vi "Display Item Info.vi"(8 "error in (no error)":errorcluster, 9 "Config":T1, 10 "Control References":T5, 11 "VI in":refnum<class "VI.lvclass">) -> (0 "error out":errorcluster, 3 "VI out":refnum<class "VI.lvclass">)   [LabVIEW 2020, in "VI Properties Editor.lvlib" / "VI.lvclass"]
doc: "Displays the data of <B>VI in</B> to the controls identified by <B>Control References</B>, taking into account <B>Config</B>."
uses:
  VI.lvclass
  C:/Users/acasalen/Documents/LabVIEW Data/Projects/VI-Properties-Editor/source/Classes/Item/Item.lvclass
  <vilib>/LabVIEW Icon API/lv_icon/Classes/Icon/Icon.lvclass
  Control/Control.lvclass
  VI Properties Editor.lvlib
  <vilib>/LabVIEW Icon API/LabVIEW Icon API.lvlib
  CTLs/Main References.ctl
  CTLs/Filter Column.ctl
  CTLs/Filter Type.ctl
  CTLs/Filter Info.ctl
  CTLs/Config.ctl
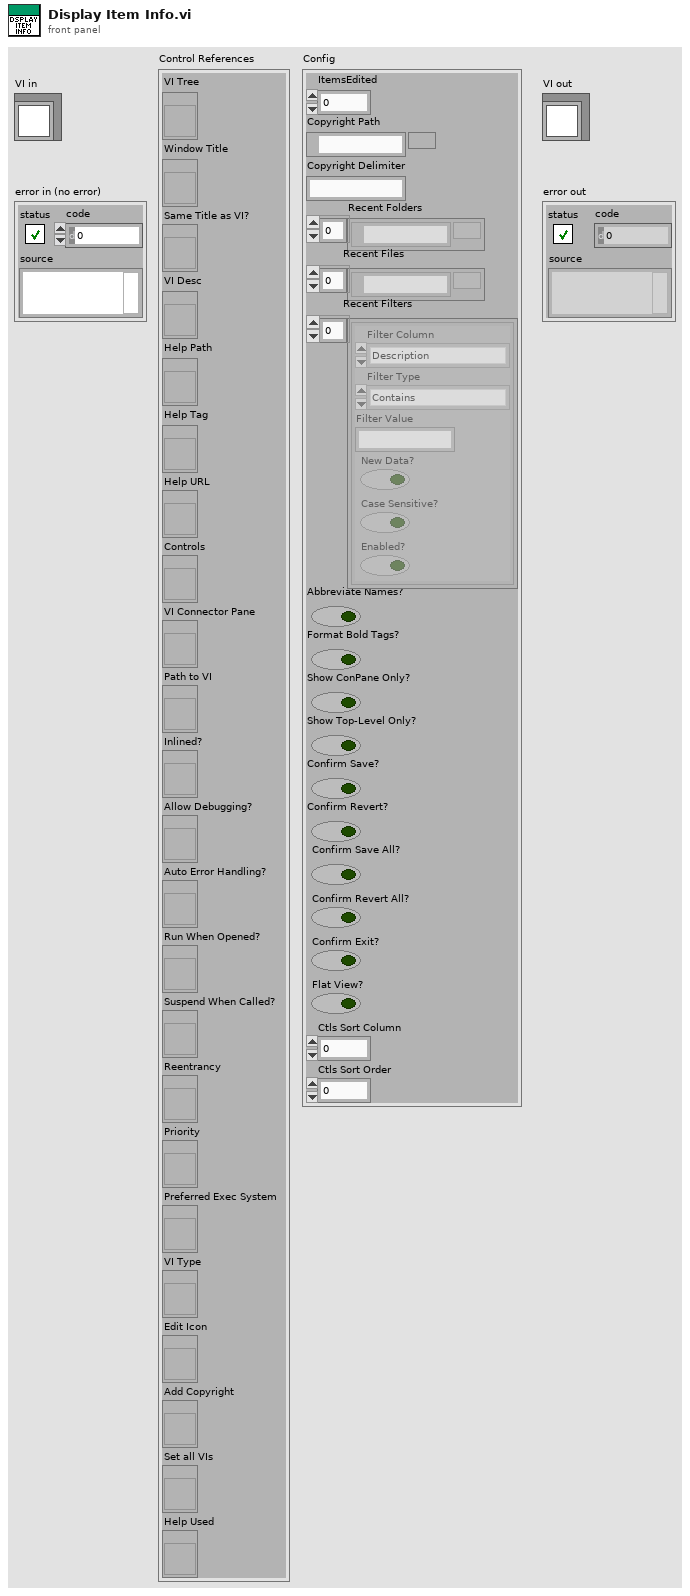
[diagram p1: front panel]
types:
  T1 = typedef "VI Properties Editor.lvlib/Config.ctl" = cluster{"ItemsEdited":u32, "Copyright Path":path, "Copyright Delimiter":string, "Recent Folders":path[], "Recent Files":path[], "Recent Filters":T2[], "Abbreviate Names?":bool, "Format Bold Tags?":bool, "Show ConPane Only?":bool, "Show Top-Level Only?":bool, "Confirm Save?":bool, "Confirm Revert?":bool, "Confirm Save All?":bool, "Confirm Revert All?":bool, "Confirm Exit?":bool, "Flat View?":bool, "Ctls Sort Column":i32, "Ctls Sort Order":i32}
  T2 = typedef "VI Properties Editor.lvlib/Filter Info.ctl" = cluster{"Filter Column":T3, "Filter Type":T4, "Filter Value":string, "New Data?":bool, "Case Sensitive?":bool, "Enabled?":bool}
  T3 = typedef "VI Properties Editor.lvlib/Filter Column.ctl" = enum16{"Name", "Path", "Type", "Window Title", "Description", "Help Path", "Help Tag", "Custom Title?", "Reentrancy", "Inlined?", "Help URL", "Help Type", "Allow Debugging?", "Auto Error Handling?", "Run When Opened?", "Suspend When Called?", "Priority", "Preferred Exec Sytem", "Control Label", "Control Caption", "Control Description", "Control Tip Strip"}
  T4 = typedef "VI Properties Editor.lvlib/Filter Type.ctl" = enum16{"Contains", "Equals", "Starts with", "Ends with", "Is empty", "Does not contain", "Does not equal", "Is not empty"}
  T5 = typedef "VI Properties Editor.lvlib/Main References.ctl" = cluster{"VI Tree":refnum<vi>, "Window Title":refnum<vi>, "Same Title as VI?":refnum<vi>, "VI Desc":refnum<vi>, "Help Path":refnum<vi>, "Help Tag":refnum<vi>, "Help URL":refnum<vi>, "Controls":refnum<vi>, "VI Connector Pane":refnum<vi>, "Path to VI":refnum<vi>, "Inlined?":refnum<vi>, "Allow Debugging?":refnum<vi>, "Auto Error Handling?":refnum<vi>, "Run When Opened?":refnum<vi>, "Suspend When Called?":refnum<vi>, "Reentrancy":refnum<vi>, "Priority":refnum<vi>, "Preferred Exec System":refnum<vi>, "VI Type":refnum<vi>, "Edit Icon":refnum<vi>, "Add Copyright":refnum<vi>, "Set all VIs":refnum<vi>, "Help Used":refnum<vi>}
  T6 = typedef "imagedata.ctl" = cluster{"image type":i32, "image depth":i32, "image":u8[], "mask":u8[], "colors":u32[], "Rectangle":cluster{"left":i16, "top":i16, "right":i16, "bottom":i16}}
  T7 = enum32{"invalid execution system", "user interface", "standard", "instrument i/o", "data acquisition", "other 1", "other 2", "same as caller"}
  T8 = enum32{"invalid VI type", "Standard VI", "Control VI", "Global VI", "Polymorphic VI", "Configuration VI", "SubSystem", "Facade VI", "Method VI", "Statechart Diagram VI"}
  T9 = enum32{"invalid priority", "background priority", "normal priority", "above normal priority", "high priority", "time critical priority", "subroutine"}
  T10 = enum16{"Share clones between instances", "Preallocate clone for each instance"}
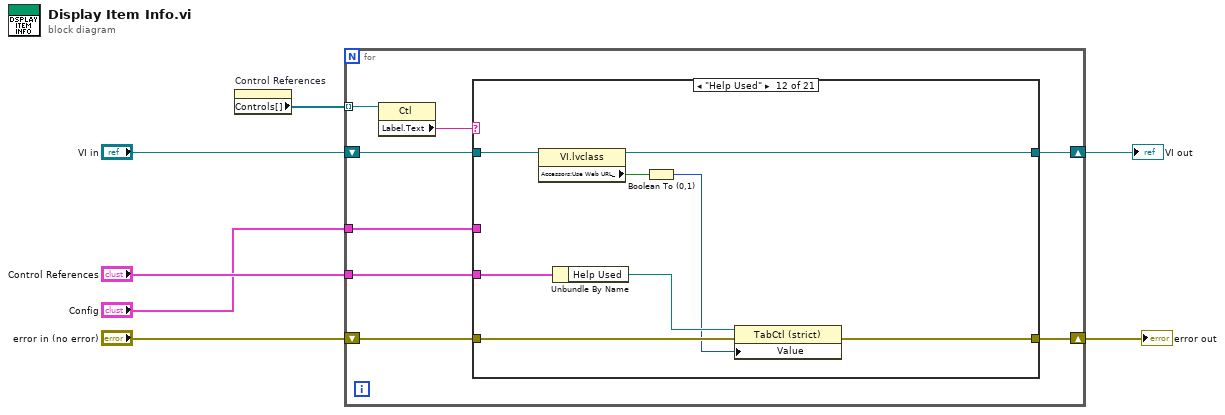
[diagram p0: block diagram]
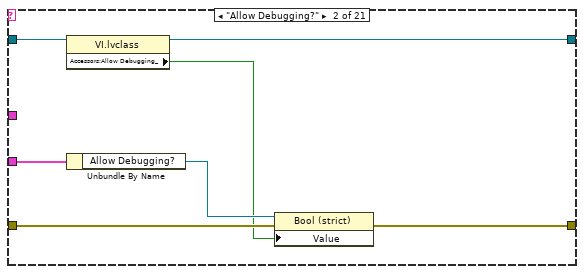
[diagram p3: hidden frame]
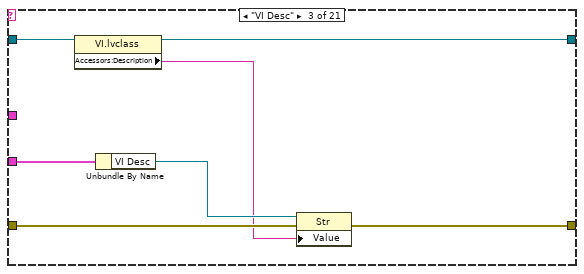
[diagram p4: hidden frame]
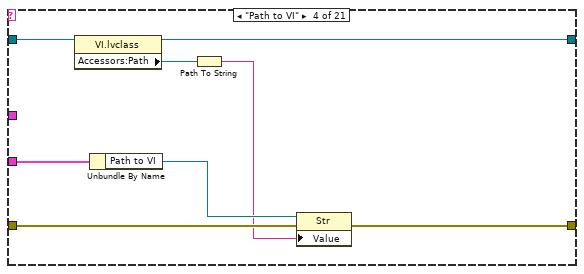
[diagram p5: hidden frame]
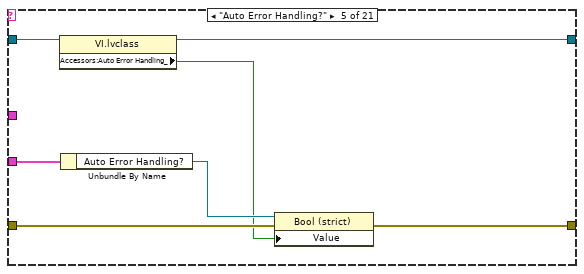
[diagram p6: hidden frame]
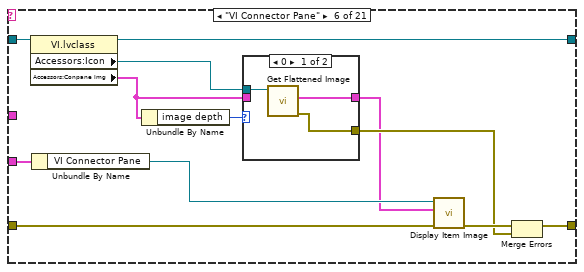
[diagram p7: hidden frame]
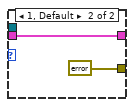
[diagram p8: hidden frame]
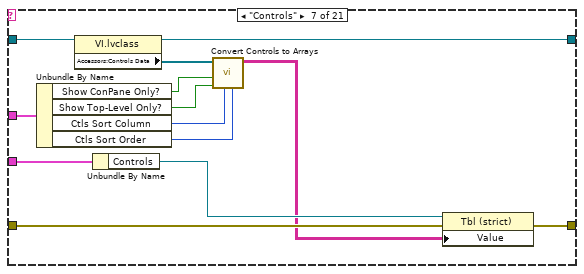
[diagram p9: hidden frame]
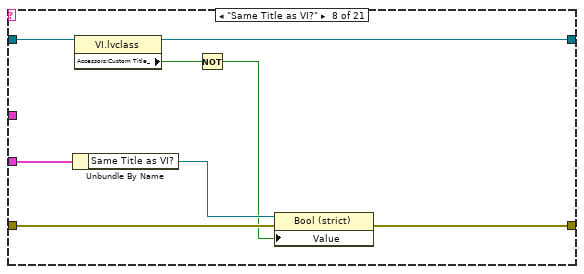
[diagram p10: hidden frame]
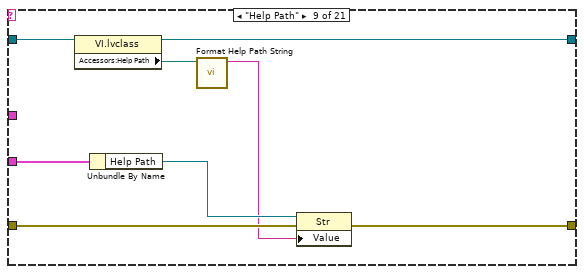
[diagram p11: hidden frame]
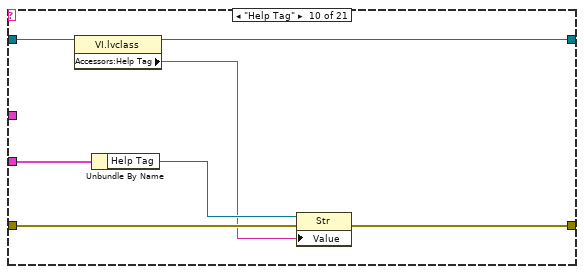
[diagram p12: hidden frame]
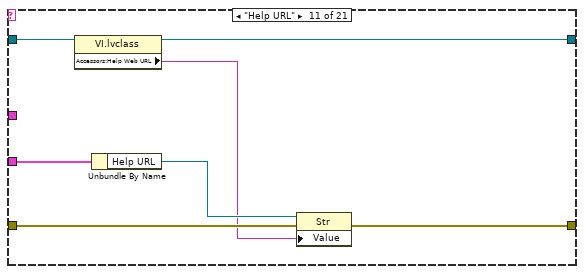
[diagram p13: hidden frame]
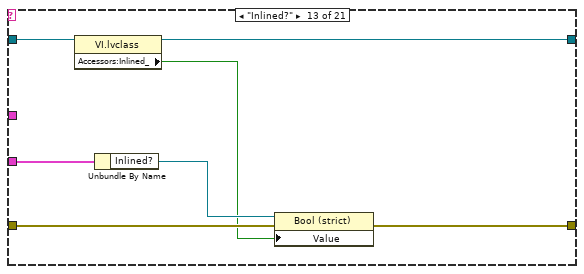
[diagram p14: hidden frame]
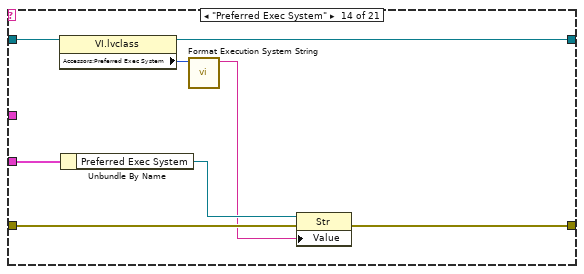
[diagram p15: hidden frame]
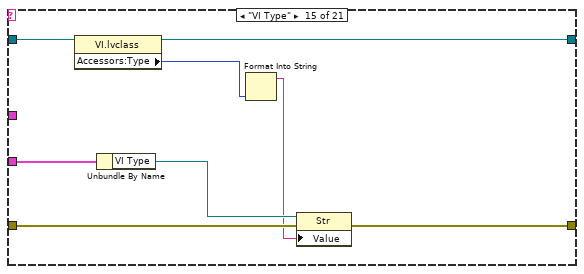
[diagram p16: hidden frame]
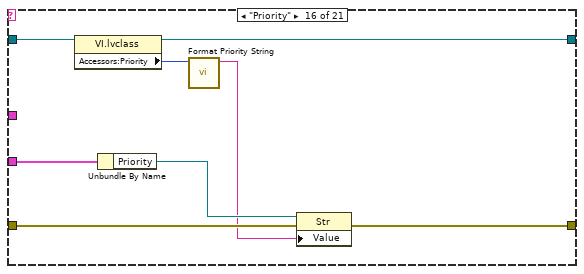
[diagram p17: hidden frame]
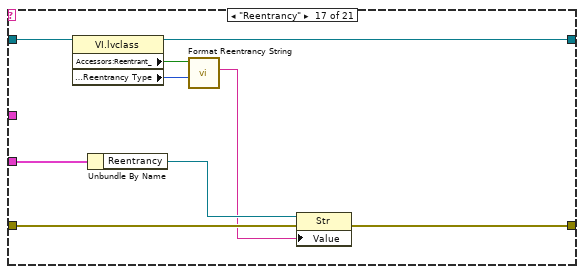
[diagram p18: hidden frame]
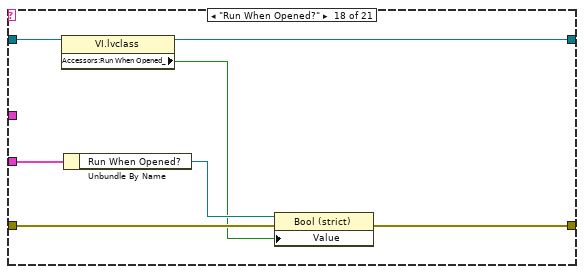
[diagram p19: hidden frame]
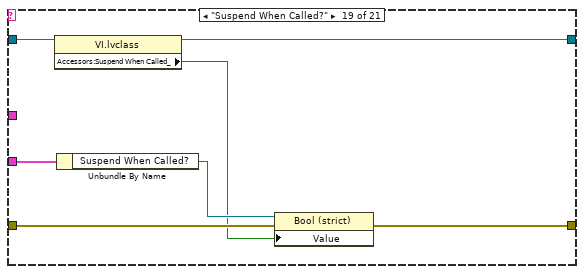
[diagram p20: hidden frame]
diagram:
  n1 = property on="Control References" class="Clust (strict)"() -> ("Controls[]"=w5:refnum<vi>[])  [unwired: 2 in, 2 out]
  n2 = for {
    shift-right: [w14] -> w6
    shift-left: "VI in" -> [w15]
    tunnel: w5 -> [w12] mode=indexing
    shift-right: [w10] -> w2
    shift-left: "error in (no error)" -> [w13]
    tunnel: "Control References" -> [w11]
    tunnel: "Config" -> [w9]
    n3 = property class="Ctl"(reference=w12) -> ("Label.Text"=w8:string)  [unwired: 1 in, 2 out]
    n4 = case shown="\"Help Used\"" w8 {
      tunnel: w15 -> [w17 w24 w31 w39 w46 w58 w76 w84 w92 w99 w106 w114 w121 w129 w137 w145 w154 w161 w168 w175 w177]
      tunnel: [w17 w23 w30 w38 w45 w57 w75 w83 w91 w98 w105 w113 w120 w128 w136 w144 w153 w160 w167 w174 w177] -> w14
      tunnel: w13 -> [w16 w20 w27 w35 w42 w49 w72 w80 w88 w95 w102 w110 w117 w125 w133 w141 w150 w157 w164 w171 w176]
      tunnel: w11 -> [_ w22 w29 w37 w44 w56 w74 w82 w90 w97 w104 w112 w119 w127 w135 w143 w152 w159 w166 w173 _]
      tunnel: [w16 w18 w25 w33 w40 w51 w71 w79 w87 w94 w101 w109 w116 w124 w132 w140 w149 w156 w163 w170 w176] -> w10
      tunnel: w9 -> [_ _ _ _ _ _ w69 _ _ _ _ _ _ _ _ _ _ _ _ _ _]
      frame Default {
      }
      frame "Allow Debugging?" {
        n5 = property class="VI.lvclass"(reference=w24) -> (reference out=w23:refnum<class "VI.lvclass">, "Accessors:Allow Debugging_"=w19:bool)  [unwired: 1 in, 1 out]
        n6 = Unbundle By Name(w22) -> ("Allow Debugging?"=w21:refnum<vi>)
        n7 = property class="Bool (strict)"(reference=w21, error in=w20, "Value"=w19) -> (error out=w18:errorcluster)  [unwired: 1 out]
      }
      frame "VI Desc" {
        n8 = property class="VI.lvclass"(reference=w31) -> (reference out=w30:refnum<class "VI.lvclass">, "Accessors:Description"=w26:string)  [unwired: 1 in, 1 out]
        n9 = Unbundle By Name(w29) -> ("VI Desc"=w28:refnum<vi>)
        n10 = property class="Str"(reference=w28, error in=w27, "Value"=w26) -> (error out=w25:errorcluster)  [unwired: 1 out]
      }
      frame "Path to VI" {
        n11 = property class="VI.lvclass"(reference=w39) -> (reference out=w38:refnum<class "VI.lvclass">, "Accessors:Path"=w34:path)  [unwired: 1 in, 1 out]
        n12 = Unbundle By Name(w37) -> ("Path to VI"=w36:refnum<vi>)
        n13 = Path To String(path=w34) -> (string=w32:string)
        n14 = property class="Str"(reference=w36, error in=w35, "Value"=w32) -> (error out=w33:errorcluster)  [unwired: 1 out]
      }
      frame "Auto Error Handling?" {
        n15 = property class="VI.lvclass"(reference=w46) -> (reference out=w45:refnum<class "VI.lvclass">, "Accessors:Auto Error Handling_"=w41:bool)  [unwired: 1 in, 1 out]
        n16 = Unbundle By Name(w44) -> ("Auto Error Handling?"=w43:refnum<vi>)
        n17 = property class="Bool (strict)"(reference=w43, error in=w42, "Value"=w41) -> (error out=w40:errorcluster)  [unwired: 1 out]
      }
      frame "VI Connector Pane" {
        n18 = property class="VI.lvclass"(reference=w58) -> (reference out=w57:refnum<class "VI.lvclass">, "Accessors:Icon"=w53:refnum<class "Icon.lvclass">, "Accessors:Conpane Img"=w52:T6)  [unwired: 1 in, 1 out]
        n19 = Unbundle By Name(w56) -> ("VI Connector Pane"=w48:refnum<vi>)
        n20 = Unbundle By Name(w52) -> ("image depth"=w54:i32)
        n21 = case shown="0" w54 {
          tunnel: w53 -> [w61 _]
          tunnel: w52 -> [_ w63]
          tunnel: [w60 errorcluster {"status"=FALSE, "code"=0, "source"=""} ("error out")] -> w50
          tunnel: [w59 w63] -> w47
          frame 0 {
            n22 = call <vilib>:"Get Flattened Image.vi"("lv_icon.lvlib:Icon.lvclass in"=w61) -> ("error out"=w60:errorcluster, "Color Image"=w59:T6)  [unwired: 7 in, 2 out]
          }
          frame 1, Default {
          }
        }
        n23 = call "Display Item Image.vi"("error in (no error)"=w49, "Color Image"=w47, "2D Picture Ref"=w48) -> ("error out"=w55:errorcluster)  [unwired: 8 in]
        n24 = Merge Errors(w55, w50) -> (w51:errorcluster)
      }
      frame "Controls" {
        n25 = Unbundle By Name(w69) -> ("Show ConPane Only?"=w68:bool, "Show Top-Level Only?"=w67:bool, "Ctls Sort Column"=w66:i32, "Ctls Sort Order"=w65:i32)
        n26 = property class="VI.lvclass"(reference=w76) -> (reference out=w75:refnum<class "VI.lvclass">, "Accessors:Controls Data"=w70:refnum<class "Control.lvclass">[])  [unwired: 1 in, 1 out]
        n27 = Unbundle By Name(w74) -> ("Controls"=w73:refnum<vi>)
        n28 = call "Convert Controls to Arrays.vi"("Sort Order"=w65, "Sort Column"=w66, "Top-Level Only?"=w67, "ConPane Only?"=w68, "Controls Data"=w70) -> ("Control Array"=w64:string[][])  [unwired: 6 in]
        n29 = property class="Tbl (strict)"(reference=w73, error in=w72, "Value"=w64) -> (error out=w71:errorcluster)  [unwired: 1 out]
      }
      frame "Same Title as VI?" {
        n30 = Unbundle By Name(w82) -> ("Same Title as VI?"=w81:refnum<vi>)
        n31 = property class="VI.lvclass"(reference=w84) -> (reference out=w83:refnum<class "VI.lvclass">, "Accessors:Custom Title_"=w78:bool)  [unwired: 1 in, 1 out]
        n32 = Not(x=w78) -> (.not. x?=w77:bool)
        n33 = property class="Bool (strict)"(reference=w81, error in=w80, "Value"=w77) -> (error out=w79:errorcluster)  [unwired: 1 out]
      }
      frame "Help Path" {
        n34 = property class="VI.lvclass"(reference=w92) -> (reference out=w91:refnum<class "VI.lvclass">, "Accessors:Help Path"=w85:path)  [unwired: 1 in, 1 out]
        n35 = Unbundle By Name(w90) -> ("Help Path"=w89:refnum<vi>)
        n36 = call "Format Help Path String.vi"("Help Path"=w85) -> ("Help Path String"=w86:string)  [unwired: 10 in]
        n37 = property class="Str"(reference=w89, error in=w88, "Value"=w86) -> (error out=w87:errorcluster)  [unwired: 1 out]
      }
      frame "Help Tag" {
        n38 = property class="VI.lvclass"(reference=w99) -> (reference out=w98:refnum<class "VI.lvclass">, "Accessors:Help Tag"=w93:string)  [unwired: 1 in, 1 out]
        n39 = Unbundle By Name(w97) -> ("Help Tag"=w96:refnum<vi>)
        n40 = property class="Str"(reference=w96, error in=w95, "Value"=w93) -> (error out=w94:errorcluster)  [unwired: 1 out]
      }
      frame "Help URL" {
        n41 = property class="VI.lvclass"(reference=w106) -> (reference out=w105:refnum<class "VI.lvclass">, "Accessors:Help Web URL"=w100:string)  [unwired: 1 in, 1 out]
        n42 = Unbundle By Name(w104) -> ("Help URL"=w103:refnum<vi>)
        n43 = property class="Str"(reference=w103, error in=w102, "Value"=w100) -> (error out=w101:errorcluster)  [unwired: 1 out]
      }
      frame "Help Used" {
        n44 = property class="VI.lvclass"(reference=w114) -> (reference out=w113:refnum<class "VI.lvclass">, "Accessors:Use Web URL_"=w108:bool)  [unwired: 1 in, 1 out]
        n45 = Unbundle By Name(w112) -> ("Help Used"=w111:refnum<vi>)
        n46 = Boolean To (0,1)(Boolean=w108) -> (0, 1=w107:i16)
        n47 = property class="TabCtl (strict)"(reference=w111, error in=w110, "Value"=w107) -> (error out=w109:errorcluster)  [unwired: 1 out]
      }
      frame "Inlined?" {
        n48 = property class="VI.lvclass"(reference=w121) -> (reference out=w120:refnum<class "VI.lvclass">, "Accessors:Inlined_"=w115:bool)  [unwired: 1 in, 1 out]
        n49 = Unbundle By Name(w119) -> ("Inlined?"=w118:refnum<vi>)
        n50 = property class="Bool (strict)"(reference=w118, error in=w117, "Value"=w115) -> (error out=w116:errorcluster)  [unwired: 1 out]
      }
      frame "Preferred Exec System" {
        n51 = property class="VI.lvclass"(reference=w129) -> (reference out=w128:refnum<class "VI.lvclass">, "Accessors:Preferred Exec System"=w123:T7)  [unwired: 1 in, 1 out]
        n52 = Unbundle By Name(w127) -> ("Preferred Exec System"=w126:refnum<vi>)
        n53 = call "Format Execution System String.vi"("Preferred Exec System"=w123) -> ("Preferred Exec System String"=w122:string)  [unwired: 10 in]
        n54 = property class="Str"(reference=w126, error in=w125, "Value"=w122) -> (error out=w124:errorcluster)  [unwired: 1 out]
      }
      frame "VI Type" {
        n55 = property class="VI.lvclass"(reference=w137) -> (reference out=w136:refnum<class "VI.lvclass">, "Accessors:Type"=w131:T8)  [unwired: 1 in, 1 out]
        n56 = Unbundle By Name(w135) -> ("VI Type"=w134:refnum<vi>)
        n57 = Format Into String(w131) -> (resulting string=w130:string)  [unwired: 3 in, 1 out]
        n58 = property class="Str"(reference=w134, error in=w133, "Value"=w130) -> (error out=w132:errorcluster)  [unwired: 1 out]
      }
      frame "Priority" {
        n59 = property class="VI.lvclass"(reference=w145) -> (reference out=w144:refnum<class "VI.lvclass">, "Accessors:Priority"=w139:T9)  [unwired: 1 in, 1 out]
        n60 = Unbundle By Name(w143) -> ("Priority"=w142:refnum<vi>)
        n61 = call "Format Priority String.vi"("Priority"=w139) -> ("Priority String"=w138:string)  [unwired: 10 in]
        n62 = property class="Str"(reference=w142, error in=w141, "Value"=w138) -> (error out=w140:errorcluster)  [unwired: 1 out]
      }
      frame "Reentrancy" {
        n63 = property class="VI.lvclass"(reference=w154) -> (reference out=w153:refnum<class "VI.lvclass">, "Accessors:Reentrant_"=w148:bool, "Accessors:Reentrancy Type"=w146:T10)  [unwired: 1 in, 1 out]
        n64 = Unbundle By Name(w152) -> ("Reentrancy"=w151:refnum<vi>)
        n65 = call "Format Reentrancy String.vi"("Reentrancy Type"=w146, "Reentrant?"=w148) -> ("Reentrancy String"=w147:string)  [unwired: 9 in]
        n66 = property class="Str"(reference=w151, error in=w150, "Value"=w147) -> (error out=w149:errorcluster)  [unwired: 1 out]
      }
      frame "Run When Opened?" {
        n67 = property class="VI.lvclass"(reference=w161) -> (reference out=w160:refnum<class "VI.lvclass">, "Accessors:Run When Opened_"=w155:bool)  [unwired: 1 in, 1 out]
        n68 = Unbundle By Name(w159) -> ("Run When Opened?"=w158:refnum<vi>)
        n69 = property class="Bool (strict)"(reference=w158, error in=w157, "Value"=w155) -> (error out=w156:errorcluster)  [unwired: 1 out]
      }
      frame "Suspend When Called?" {
        n70 = property class="VI.lvclass"(reference=w168) -> (reference out=w167:refnum<class "VI.lvclass">, "Accessors:Suspend When Called_"=w162:bool)  [unwired: 1 in, 1 out]
        n71 = Unbundle By Name(w166) -> ("Suspend When Called?"=w165:refnum<vi>)
        n72 = property class="Bool (strict)"(reference=w165, error in=w164, "Value"=w162) -> (error out=w163:errorcluster)  [unwired: 1 out]
      }
      frame "Window Title" {
        n73 = property class="VI.lvclass"(reference=w175) -> (reference out=w174:refnum<class "VI.lvclass">, "Accessors:Window Title"=w169:string)  [unwired: 1 in, 1 out]
        n74 = Unbundle By Name(w173) -> ("Window Title"=w172:refnum<vi>)
        n75 = property class="Str"(reference=w172, error in=w171, "Value"=w169) -> (error out=w170:errorcluster)  [unwired: 1 out]
      }
      frame "VI Tree" {
        # "Nothing currently done to set the value of the VI Tree programmatically"
      }
    }
  }
  "error out" <- w2
  "VI out" <- w6
